vi "Get TableItem.vi"(8 "error in (no error)":errorcluster, 11 "ScriptDatabase in":refnum<class "ScriptDatabase.lvclass">) -> (0 "error out":errorcluster, 2 "TableItem":T1[](array[typedef])=[{"column name"="ID", "data type"=enum."Single (SGL)", "size"=0, "allow null?"=TRUE}, {"column name"="FuncName", "data type"=enum."String", "size"=0, "allow null?"=FALSE}, {"column name"="FuncQuickName", "data type"=enum."String", "size"=0, "allow null?"=TRUE}, {"column name"="FunctionPath", "data type"=enum."String", "size"=0, "allow null?"=FALSE}], 3 "ScriptDatabase out":refnum<class "ScriptDatabase.lvclass">)   [LabVIEW 2015, in "ScriptDatabase.lvclass"]
uses:
  ScriptDatabase.lvclass
  <vilib>/addons/database/Auxilliary.llb/DB Tools Column Info.ctl
  <vilib>/addons/database/Auxilliary.llb/DB Tools DataTypes.ctl
  ScriptDatabase.lvclass/ScriptDatabase.ctl
  <vilib>/addons/database/NI_Database_API.lvlib
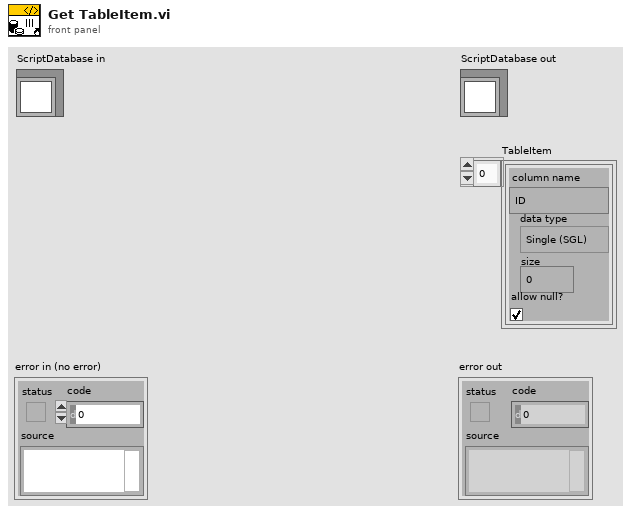
[diagram p1: front panel]
types:
  T1 = typedef "NI_Database_API.lvlib/DB Tools Column Info.ctl" = cluster{"column name":string, "data type":T2, "size":i32, "allow null?":bool}
  T2 = typedef "NI_Database_API.lvlib/DB Tools DataTypes.ctl" = enum16{"String", "Long (I32)", "Single (SGL)", "Double (DBL)", "Date/Time", "Binary"}
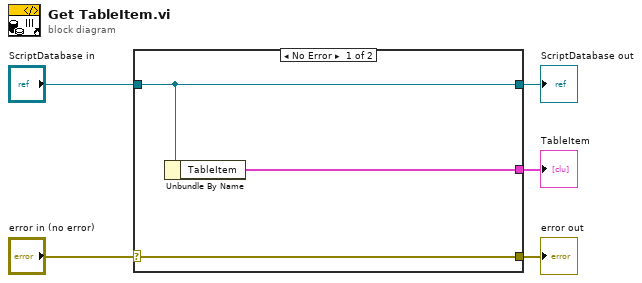
[diagram p0: block diagram]
diagram:
  n1 = case shown="No Error" "error in (no error)" {
    selector: "error in (no error)" -> [w8 w9]
    tunnel: [w8 w9] -> w4
    tunnel: [w7 w10] -> w2
    tunnel: "ScriptDatabase in" -> [w7 w10]
    tunnel: [w6 _] -> w1
    frame No Error {
      n2 = Unbundle By Name(w7) -> ("TableItem"=w6:T1[])
    }
    frame Error {
    }
  }
  "error out" <- w4
  "ScriptDatabase out" <- w2
  "TableItem" <- w1
